vi "gyro -- async pll monitor V1.vi"(8 "pll engine pair IN":T6, 11 "pll monitor event pair IN":T6) -> ()   [LabVIEW 2020]
uses:
  lorentzian.ctl
  circle corners.ctl
  show-win- control.ctl
  server talk-to-back pair.ctl
  server talkback message type.ctl
  server talkto message type.ctl
  pll internal user event action.ctl
  launch items list.ctl
  que event bag action.ctl
  agregator -- action.ctl
  publisher action.ctl
  cursor action.ctl
  four-corner circle transformation.ctl
  draw a circle.vi
  draw a complex arrow.vi
  Q -- check range -- i -- real.vi
  generate linear region.vi
  draw a complex line.vi
  Q - not nan -- real.vi
panel:
  out "slow G (Hz)":dbl=24.16832544290019 format="%#.4f"
  out "slow f (Hz)":dbl=46363.51241324636 format="%#.11f"
  in  "all 3":T1(tab)
  in  "Reset lore :q":bool
  in  "Tab Control":enum32{"PID", "hist", "params"}(tab)
  out "Plot: complex plane":cluster{dbl[], dbl[]}[](graph)
  out "Plot: complex- hist":cluster{dbl[], dbl[]}[](graph)=[{[-9.526305317469014e-05, -9.526305317469014e-05, -9.526305317469014e-05, -9.526305317469014e-05, -9.526305317469014e-05, -9.526305317469014e-05, -9.526305317469014e-05, -9.526305317469014e-05, -9.526305317469014e-05, -9.526305317469014e-05, -9.526305317469014e-05, -9.526305317469014e-05, -9.496573362823372e-05, -9.462272279446522e-05, -9.456910422622903e-05, -9.455599564968666e-05, -9.455599564968666e-05, -9.455599564968666e-05, -9.455599564968666e-05, -9.455599564968666e-05, -9.455599564968666e-05, -9.530610879315279e-05, -9.530610879315279e-05, -9.634850628222362e-05, -9.634850628222362e-05, -9.634850628222362e-05, -9.634850628222362e-05, -9.634850628222362e-05, -9.634850628222362e-05, -9.634850628222362e-05, -0.00010067313796781224, -0.00010168181201432396, -0.00010343088718200523, -0.00010398871218266516, -0.00010398871218266516, -0.00010398871218266516, -0.00010398871218266516, -0.00010398871218266516, -0.00010398871218266516, -0.00010398871218266516, -0.00010398871218266516, -0.00010398871218266516, -0.00011483545491618031, -0.00011483545491618031, -0.00011483545491618031, -0.00011483545491618031, -0.00011483545491618031, -0.00011483545491618031, -0.00011483545491618031, -0.00011483545491618031], [7.970920146417072e-05, 7.970920146417072e-05, 7.970920146417072e-05, 7.970920146417072e-05, 7.970920146417072e-05, 7.970920146417072e-05, 7.970920146417072e-05, 7.970920146417072e-05, 7.970920146417072e-05, 7.970920146417072e-05, 7.970920146417072e-05, 7.970920146417072e-05, 7.992857617299889e-05, 8.004706678063113e-05, 8.0440222108718e-05, 8.032807976592085e-05, 8.032807976592085e-05, 8.032807976592085e-05, 8.032807976592085e-05, 8.032807976592085e-05, 8.032807976592085e-05, 8.12855651877623e-05, 8.12855651877623e-05, 8.097547218826884e-05, 8.097547218826884e-05, 8.097547218826884e-05, 8.097547218826884e-05, 8.097547218826884e-05, 8.097547218826884e-05, 8.097547218826884e-05, 8.470777605978184e-05, 8.527717057334149e-05, 8.650804581518505e-05, 8.815252786351578e-05, 8.815252786351578e-05, 8.815252786351578e-05, 8.815252786351578e-05, 8.815252786351578e-05, 8.815252786351578e-05, 8.815252786351578e-05, 8.815252786351578e-05, 8.815252786351578e-05, 9.872168338494033e-05, 9.872168338494033e-05, 9.872168338494033e-05, 9.872168338494033e-05, 9.872168338494033e-05, 9.872168338494033e-05, 9.872168338494033e-05, 9.872168338494033e-05]}, {[3.818876044553316e-06, 3.7612071619776832e-06, 3.588301685066841e-06, 3.300462948780953e-06, 2.8981959200717497e-06, 2.3822063119988216e-06, 1.7533993456691853e-06, 1.0128781621718285e-06, 1.6194188729338013e-07, -7.979166475899173e-07, -1.8650135244457675e-06, -3.037476692750206e-06, -4.313249253700366e-06, -5.690093068713917e-06, -7.1655926858846405e-06, -8.737159577505894e-06, -1.0402036681227744e-05, -1.2157303236881222e-05, -1.3999879910484142e-05, -1.592653419643923e-05, -1.79338860884474e-05, -2.001841400918731e-05, -2.2176460988358644e-05, -2.440424107825063e-05, -2.6697845995580853e-05, -2.9053251977952116e-05, -3.146632684289902e-05, -3.3932837237140076e-05, -3.6448456063317944e-05, -3.900877007119849e-05, -4.1609287600011325e-05, -4.4245446458349125e-05, -4.691262192780158e-05, -4.9606134876282945e-05, -5.232125996681972e-05, -5.505323394739742e-05, -5.779726400732312e-05, -6.054853618544401e-05, -6.330222381547109e-05, -6.605349599359198e-05, -6.879752605351768e-05, -7.152950003409537e-05, -7.424462512463216e-05, -7.693813807311352e-05, -7.960531354256597e-05, -8.224147240090377e-05, -8.484198992971662e-05, -8.740230393759715e-05, -8.991792276377502e-05, -9.238443315801609e-05, -9.479750802296298e-05, -9.715291400533426e-05, -9.944651892266448e-05, -0.00010167429901255647, -0.00010383234599172779, -0.00010591687391246771, -0.00010792422580447587, -0.00010985088009043097, -0.00011169345676403388, -0.00011344872331968736, -0.00011511360042340923, -0.00011668516731503045, -0.00011816066693220119, -0.00011953751074721475, -0.0001208132833081649, -0.00012198574647646935, -0.0001230528433533252, -0.0001240127018882085, -0.00012486363816308695, -0.0001256041593465843, -0.00012623296631291396, -0.00012674895592098688, -0.00012715122294969607, -0.00012743906168598198, -0.00012761196716289282, -0.00012766963604546842, -0.00012761196716289282, -0.00012743906168598198, -0.00012715122294969607, -0.00012674895592098688, -0.00012623296631291396, -0.00012560415934658432, -0.00012486363816308695, -0.00012401270188820853, -0.00012305284335332523, -0.00012198574647646936, -0.00012081328330816493, -0.00011953751074721476, -0.00011816066693220122, -0.00011668516731503051, -0.00011511360042340925, -0.00011344872331968739, -0.0001116934567640339, -0.000109850880090431, -0.00010792422580447591, -0.00010591687391246773, -0.00010383234599172784, -0.0001016742990125565, -9.944651892266452e-05, -9.715291400533429e-05, -9.479750802296303e-05, -9.238443315801612e-05, -8.991792276377506e-05, -8.740230393759719e-05, -8.484198992971665e-05, -8.22414724009038e-05, -7.9605313542566e-05, -7.69381380731136e-05, -7.424462512463222e-05, -7.152950003409544e-05, -6.879752605351773e-05, -6.605349599359204e-05, -6.330222381547115e-05, -6.054853618544405e-05, -5.779726400732316e-05, -5.505323394739747e-05, -5.232125996681976e-05, -4.960613487628297e-05, -4.691262192780161e-05, -4.424544645834915e-05, -4.160928760001134e-05, -3.900877007119856e-05, -3.644845606331801e-05, -3.393283723714014e-05, -3.146632684289907e-05, -2.905325197795217e-05, -2.66978459955809e-05, -2.4404241078250677e-05, -2.2176460988358678e-05, -2.0018414009187342e-05, -1.7933886088447427e-05, -1.5926534196439257e-05, -1.3999879910484162e-05, -1.2157303236881242e-05, -1.0402036681227757e-05, -8.7371595775059e-06, -7.165592685884681e-06, -5.690093068713951e-06, -4.3132492537004e-06, -3.037476692750233e-06, -1.8650135244457946e-06, -7.979166475899309e-07, 1.6194188729336657e-07, 1.012878162171815e-06, 1.7533993456691853e-06, 2.3822063119988216e-06, 2.8981959200717497e-06, 3.300462948780953e-06, 3.588301685066841e-06, 3.7612071619776832e-06], [0.00013328633245229232, 0.00013603941615311703, 0.0001387876700096264, 0.0001415262726506931, 0.00014425041963670132, 0.00014695533188816622, 0.0001496362640698634, 0.00015228851291575925, 0.00015490742548013788, 0.00015748840730044888, 0.00016002693045755594, 0.0001625185415192455, 0.0001649588693530602, 0.00016734363279475065, 0.00016966864815889197, 0.00017192983657849, 0.00017412323116069973, 0.00017624498394610346, 0.00017829137265933922, 0.00018025880723923637, 0.00018214383613700304, 0.00018394315237141542, 0.0001856535993303866, 0.00018727217630873675, 0.00018879604377244967, 0.0001902225283401804, 0.0001915491274732744, 0.0001927735138660708, 0.00019389353952878736, 0.00019490723955582442, 0.00019581283557287696, 0.00019660873885680747, 0.00019729355312280615, 0.00019786607697394902, 0.00019832530600885628, 0.0001986704345837536, 0.00019890085722584514, 0.00019901616969551854, 0.00019901616969551854, 0.00019890085722584514, 0.0001986704345837536, 0.00019832530600885628, 0.00019786607697394902, 0.00019729355312280615, 0.00019660873885680747, 0.00019581283557287696, 0.00019490723955582442, 0.0001938935395287874, 0.00019277351386607082, 0.0001915491274732744, 0.0001902225283401804, 0.00018879604377244967, 0.00018727217630873675, 0.00018565359933038662, 0.00018394315237141545, 0.00018214383613700307, 0.00018025880723923637, 0.00017829137265933922, 0.00017624498394610348, 0.00017412323116069973, 0.00017192983657849, 0.000169668648158892, 0.00016734363279475065, 0.00016495886935306023, 0.00016251854151924552, 0.00016002693045755596, 0.0001574884073004489, 0.00015490742548013788, 0.00015228851291575928, 0.00014963626406986344, 0.00014695533188816625, 0.00014425041963670135, 0.00014152627265069312, 0.0001387876700096264, 0.00013603941615311706, 0.00013328633245229235, 0.00013053324875146764, 0.0001277849948949583, 0.00012504639225389158, 0.00012232224526788335, 0.00011961733301641843, 0.00011693640083472126, 0.00011428415198882542, 0.0001116652394244468, 0.00010908425760413579, 0.00010654573444702874, 0.00010405412338533918, 0.00010161379555152444, 9.922903210983402e-05, 9.69040167456927e-05, 9.464282832609468e-05, 9.244943374388495e-05, 9.032768095848119e-05, 8.828129224524545e-05, 8.631385766534829e-05, 8.44288287675816e-05, 8.262951253316924e-05, 8.091906557419806e-05, 7.930048859584792e-05, 7.777662113213499e-05, 7.635013656440427e-05, 7.502353743131027e-05, 7.379915103851385e-05, 7.267912537579728e-05, 7.166542534876021e-05, 7.07598293317077e-05, 6.996392604777719e-05, 6.927911178177851e-05, 6.870658793063563e-05, 6.824735889572837e-05, 6.790223032083105e-05, 6.76718076787395e-05, 6.755649520906611e-05, 6.755649520906611e-05, 6.76718076787395e-05, 6.790223032083104e-05, 6.824735889572836e-05, 6.870658793063562e-05, 6.92791117817785e-05, 6.996392604777719e-05, 7.075982933170768e-05, 7.166542534876019e-05, 7.267912537579724e-05, 7.379915103851382e-05, 7.502353743131023e-05, 7.635013656440423e-05, 7.777662113213495e-05, 7.930048859584787e-05, 8.091906557419801e-05, 8.262951253316918e-05, 8.442882876758158e-05, 8.631385766534825e-05, 8.828129224524542e-05, 9.032768095848116e-05, 9.244943374388492e-05, 9.464282832609465e-05, 9.690401674569261e-05, 9.922903210983394e-05, 0.00010161379555152437, 0.00010405412338533911, 0.00010654573444702866, 0.00010908425760413571, 0.00011166523942444672, 0.00011428415198882535, 0.0001169364008347212, 0.00011961733301641839, 0.0001223222452678833, 0.00012504639225389153, 0.00012778499489495826, 0.0001305332487514676]}, {[3.628480178228017e-06, -3.271926156370463e-06, -1.0172332490968943e-05, -1.7072738825567422e-05, -2.3973145160165903e-05, -3.087355149476438e-05, -3.777395782936286e-05, -4.467436416396134e-05, -5.157477049855982e-05, -5.8475176833158303e-05, -6.537558316775678e-05, -7.227598950235527e-05, -7.917639583695374e-05, -8.607680217155223e-05, -9.29772085061507e-05, -9.987761484074919e-05, -0.00010677802117534766, -0.00011367842750994615, -0.00012057883384454462, -0.00012747924017914312], [0.00013828619430891303, 0.0001377598930608477, 0.00013723359181278235, 0.00013670729056471703, 0.00013618098931665167, 0.00013565468806858635, 0.000135128386820521, 0.00013460208557245567, 0.00013407578432439034, 0.00013354948307632499, 0.00013302318182825966, 0.0001324968805801943, 0.00013197057933212898, 0.00013144427808406365, 0.0001309179768359983, 0.00013039167558793297, 0.00012986537433986762, 0.0001293390730918023, 0.00012881277184373694, 0.00012828647059567161]}, {[-0.00012747924017914312, -0.0001271379440244435, -0.00012679664786974387, -0.00012645535171504425, -0.00012611405556034463, -0.00012577275940564502, -0.00012543146325094537, -0.00012509016709624576, -0.00012474887094154614, -0.00012440757478684653, -0.00012406627863214688, -0.00012372498247744727, -0.00012338368632274765, -0.00012304239016804804, -0.0001227010940133484, -0.00012235979785864878, -0.00012201850170394916, -0.00012167720554924953, -0.00012133590939454991, -0.00012099461323985029], [0.00012828647059567161, 0.00012822947554103566, 0.0001281724804863997, 0.00012811548543176373, 0.00012805849037712778, 0.00012800149532249183, 0.00012794450026785587, 0.00012788750521321992, 0.00012783051015858394, 0.000127773515103948, 0.00012771652004931204, 0.0001276595249946761, 0.0001276025299400401, 0.00012754553488540416, 0.0001274885398307682, 0.00012743154477613225, 0.0001273745497214963, 0.00012731755466686032, 0.00012726055961222437, 0.00012720356455758842]}, {[-0.00012747924017914312, -0.00012715053574649993, -0.0001268218313138567, -0.0001264931268812135, -0.00012616442244857027, -0.00012583571801592707, -0.00012550701358328385, -0.00012517830915064065, -0.00012484960471799742, -0.00012452090028535422, -0.00012419219585271102, -0.0001238634914200678, -0.0001235347869874246, -0.00012320608255478137, -0.00012287737812213817, -0.00012254867368949494, -0.00012221996925685174, -0.00012189126482420853, -0.00012156256039156532, -0.0001212338559589221], [0.00012828647059567161, 0.00012839456729972132, 0.00012850266400377103, 0.0001286107607078207, 0.00012871885741187042, 0.00012882695411592013, 0.00012893505081996984, 0.00012904314752401955, 0.00012915124422806923, 0.00012925934093211894, 0.00012936743763616865, 0.00012947553434021836, 0.00012958363104426804, 0.00012969172774831775, 0.00012979982445236746, 0.00012990792115641716, 0.00013001601786046687, 0.00013012411456451655, 0.00013023221126856626, 0.00013034030797261597]}, {[-6.692524185707827e-05, -6.639894060901293e-05, -6.587263936094759e-05, -6.534633811288225e-05, -6.482003686481692e-05, -6.429373561675158e-05, -6.376743436868624e-05, -6.32411331206209e-05, -6.271483187255556e-05, -6.218853062449022e-05, -6.16622293764249e-05, -6.113592812835956e-05, -6.060962688029422e-05, -6.008332563222888e-05, -5.955702438416354e-05, -5.9030723136098205e-05, -5.8504421888032865e-05, -5.7978120639967525e-05, -5.745181939190219e-05, -5.692551814383685e-05], [0.0001988401926309779, 0.0001919397862963794, 0.00018503937996178094, 0.00017813897362718245, 0.00017123856729258396, 0.00016433816095798548, 0.00015743775462338702, 0.00015053734828878853, 0.00014363694195419004, 0.00013673653561959158, 0.0001298361292849931, 0.0001229357229503946, 0.00011603531661579613, 0.00010913491028119764, 0.00010223450394659917, 9.533409761200068e-05, 8.843369127740221e-05, 8.153328494280372e-05, 7.463287860820525e-05, 6.773247227360676e-05]}, {[-5.692551814383685e-05, -5.686852308920089e-05, -5.681152803456494e-05, -5.675453297992898e-05, -5.669753792529302e-05, -5.6640542870657065e-05, -5.658354781602111e-05, -5.6526552761385154e-05, -5.6469557706749195e-05, -5.6412562652113236e-05, -5.6355567597477284e-05, -5.6298572542841325e-05, -5.6241577488205367e-05, -5.618458243356941e-05, -5.6127587378933456e-05, -5.60705923242975e-05, -5.601359726966154e-05, -5.595660221502558e-05, -5.589960716038963e-05, -5.584261210575367e-05], [6.773247227360675e-05, 6.807376842830637e-05, 6.841506458300599e-05, 6.875636073770562e-05, 6.909765689240524e-05, 6.943895304710487e-05, 6.978024920180448e-05, 7.012154535650411e-05, 7.046284151120373e-05, 7.080413766590336e-05, 7.114543382060297e-05, 7.14867299753026e-05, 7.182802613000222e-05, 7.216932228470185e-05, 7.251061843940146e-05, 7.28519145941011e-05, 7.319321074880071e-05, 7.353450690350034e-05, 7.387580305819996e-05, 7.421709921289959e-05]}, {[-5.692551814383685e-05, -5.7033614847886554e-05, -5.7141711551936256e-05, -5.724980825598596e-05, -5.7357904960035666e-05, -5.746600166408537e-05, -5.757409836813507e-05, -5.768219507218477e-05, -5.7790291776234474e-05, -5.7898388480284176e-05, -5.8006485184333885e-05, -5.811458188838359e-05, -5.822267859243329e-05, -5.833077529648299e-05, -5.843887200053269e-05, -5.8546968704582395e-05, -5.86550654086321e-05, -5.8763162112681805e-05, -5.887125881673151e-05, -5.897935552078121e-05], [6.773247227360675e-05, 6.806117670624996e-05, 6.838988113889317e-05, 6.871858557153638e-05, 6.90472900041796e-05, 6.93759944368228e-05, 6.970469886946601e-05, 7.003340330210922e-05, 7.036210773475244e-05, 7.069081216739565e-05, 7.101951660003886e-05, 7.134822103268207e-05, 7.167692546532529e-05, 7.20056298979685e-05, 7.233433433061171e-05, 7.266303876325491e-05, 7.299174319589813e-05, 7.332044762854134e-05, 7.364915206118455e-05, 7.397785649382777e-05]}, {[-6.3712435350134095e-06, -5.318641038882734e-06, -4.266038542752058e-06, -3.213436046621383e-06, -2.160833550490707e-06, -1.1082310543600322e-06, -5.56285582293566e-08, 9.96973937901319e-07, 2.0495764340319955e-06, 3.1021789301626703e-06, 4.154781426293345e-06, 5.2073839224240215e-06, 6.259986418554696e-06, 7.312588914685373e-06, 8.365191410816048e-06, 9.417793906946724e-06, 1.04703964030774e-05, 1.1522998899208077e-05, 1.257560139533875e-05, 1.3628203891469427e-05], [0.00026939391466628416, 0.0002555931019970872, 0.00024179228932789024, 0.0002279914766586933, 0.00021419066398949631, 0.00020038985132029937, 0.00018658903865110242, 0.00017278822598190544, 0.00015898741331270847, 0.00014518660064351152, 0.00013138578797431457, 0.0001175849753051176, 0.00010378416263592065, 8.998334996672367e-05, 7.618253729752673e-05, 6.238172462832975e-05, 4.85809119591328e-05, 3.478009928993583e-05, 2.097928662073888e-05, 7.178473951541904e-06]}, {[1.3628203891469427e-05, 1.374219400074134e-05, 1.3856184110013255e-05, 1.397017421928517e-05, 1.4084164328557083e-05, 1.4198154437828998e-05, 1.4312144547100912e-05, 1.4426134656372826e-05, 1.454012476564474e-05, 1.4654114874916653e-05, 1.4768104984188567e-05, 1.4882095093460481e-05, 1.4996085202732395e-05, 1.511007531200431e-05, 1.5224065421276224e-05, 1.5338055530548138e-05, 1.5452045639820052e-05, 1.5566035749091966e-05, 1.568002585836388e-05, 1.5794015967635795e-05], [7.178473951541904e-06, 7.861066260941151e-06, 8.543658570340397e-06, 9.226250879739644e-06, 9.90884318913889e-06, 1.0591435498538137e-05, 1.1274027807937384e-05, 1.195662011733663e-05, 1.2639212426735877e-05, 1.3321804736135124e-05, 1.400439704553437e-05, 1.4686989354933617e-05, 1.5369581664332864e-05, 1.605217397373211e-05, 1.6734766283131355e-05, 1.7417358592530604e-05, 1.809995090192985e-05, 1.87825432113291e-05, 1.9465135520728344e-05, 2.014772783012759e-05]}, {[1.3628203891469427e-05, 1.3412010483370021e-05, 1.3195817075270614e-05, 1.2979623667171208e-05, 1.2763430259071802e-05, 1.2547236850972395e-05, 1.233104344287299e-05, 1.2114850034773584e-05, 1.1898656626674176e-05, 1.1682463218574771e-05, 1.1466269810475365e-05, 1.1250076402375958e-05, 1.1033882994276552e-05, 1.0817689586177147e-05, 1.0601496178077741e-05, 1.0385302769978334e-05, 1.0169109361878928e-05, 9.95291595377952e-06, 9.736722545680117e-06, 9.52052913758071e-06], [7.178473951541904e-06, 7.835882816828328e-06, 8.49329168211475e-06, 9.150700547401175e-06, 9.8081094126876e-06, 1.0465518277974024e-05, 1.1122927143260446e-05, 1.178033600854687e-05, 1.2437744873833295e-05, 1.3095153739119718e-05, 1.3752562604406142e-05, 1.4409971469692566e-05, 1.506738033497899e-05, 1.5724789200265415e-05, 1.6382198065551837e-05, 1.703960693083826e-05, 1.7697015796124686e-05, 1.8354424661411112e-05, 1.901183352669753e-05, 1.9669242391983957e-05]}]
  out "fast G (Hz)":dbl=23.890697353762498 format="%#.4f"
  in  "Reset freq :r":bool
  in  "lorentzian":T2={"A (VHz)"=0.0013732658487984977, "f (Hz)"=46364.101188801076, "G (Hz)"=24.052820242417244, "phi(rad)"=4.682548985119491, "Q"=1927.5952142625588, "Norm  Ampl"=nan, "bg (V)"=9.232975216617241e-07+0.00011328685513440606i, "4corners"={"z (-pi/2)"=-5.784846603575453e-05+5.7921940748033466e-05i, "z(inf)"=9.232975216617241e-07+0.00011328685513440606i, "z (pi/2)"=-5.444161686471088e-05+0.00017205861869182233i, "z center"=-5.61450414502327e-05+0.00011499027971992789i, "z(0)"=-0.00011321338042212712+0.00011669370430544972i, "radius"=5.709375594869902e-05}} {"bg (V)" format="%#9_9f"; "Q" format="%#9_9f"; "phi(rad)" format="%#9_9f"; "G (Hz)" format="%#9_9f"; "f (Hz)" format="%#9_9f"}
  in  "Toggle PLL :@":bool
  out "fast f (Hz)":dbl=46363.6845772732 format="%#.11f"
  in  "PLL is ON":bool
  in  "publish dt (sec)":dbl=0.01 format="%#_10f"
  in  "average time (sec)":dbl=2.0 format="%#_10f"
  in  "lorentzian -- basic":T2={"A (VHz)"=1.0, "f (Hz)"=1000.0, "G (Hz)"=3.0, "phi(rad)"=0.0, "Q"=300.0, "Norm  Ampl"=nan, "bg (V)"=0.0+0.0i, "4corners"={"z (-pi/2)"=9.277908004825974e-07+0.0007240755403629966i, "z(inf)"=2.6527949823343002e-05+0.0007477540585896028i, "z (pi/2)"=2.8494315967368497e-06+0.0007733542176124632i, "z center"=1.8886111986097237e-06+0.0007487148789877299i, "z(0)"=-2.2750727426123552e-05+0.000749675699385857i, "radius"=2.4658065287076567e-05}} {"bg (V)" format="%#9_9f"; "Q" format="%#9_9f"; "phi(rad)" format="%#9_9f"; "G (Hz)" format="%#9_9f"; "f (Hz)" format="%#9_9f"}
  in  "save lor for later":bool
  in  "reset from basic":bool
  out "zi out Im (V)":dbl=0.00011062417845810371 format="%#.8f"
  out "zi out Re (V)":dbl=-0.00011339640178767734 format="%#.8f"
  out "publish message":T4={"freq (Hz)"=46363.51241324636, "gamma (Hz)"=24.16832544290019, "Voltage (V)"=-0.00011339640178767734+0.00011062417845810371i}
  out "zi out (V)":cdb=-0.00011339640178767734+0.00011062417845810371i
  out "is publish loop stoped?":bool=TRUE
  out "window":T5={"cen (Hz)"=45496.74569300777, "win (Hz)"=29.962105514646385, "left (Hz)"=45481.76464025045, "right (Hz)"=45511.72674576509}
  out "running lorentzian out":T2={"A (VHz)"=0.0013788688861127354, "f (Hz)"=46363.6845772732, "G (Hz)"=23.890697353762498, "phi(rad)"=4.689952869394783, "Q"=1921.793640717071, "Norm  Ampl"=nan, "bg (V)"=1.441663885059972e-06+0.00010805339490546445i, "4corners"={"z (-pi/2)"=-4.886429450544085e-05+0.00017233029636879173i, "z(inf)"=1.441663885059972e-06+0.00010805339490546445i, "z (pi/2)"=-6.283523757826731e-05+5.7747436514963635e-05i, "z center"=-5.584976604185408e-05+0.00011503886644187768i, "z(0)"=-0.00011314119596876813+0.00012202433797829091i, "radius"=5.771572364318533e-05}} {"bg (V)" format="%#9_9f"; "Q" format="%#9_9f"; "phi(rad)" format="%#9_9f"; "G (Hz)" format="%#9_9f"; "f (Hz)" format="%#9_9f"}
  in  "lorentzian -- hist":T2={"A (VHz)"=0.00200421395131866, "f (Hz)"=46345.85168996005, "G (Hz)"=30.48500465115163, "phi(rad)"=-1.4946726575691582, "Q"=1520.2835695880153, "Norm  Ampl"=nan, "bg (V)"=3.628480178228017e-06+0.00013828619430891303i, "4corners"={"z (-pi/2)"=-6.692524185707827e-05+0.0001988401926309779i, "z(inf)"=3.628480178228017e-06+0.00013828619430891303i, "z (pi/2)"=-5.692551814383685e-05+6.773247227360675e-05i, "z center"=-6.192538000045756e-05+0.00013328633245229232i, "z(0)"=-0.00012747924017914312+0.00012828647059567161i, "radius"=6.574425604501088e-05}} {"bg (V)" format="%#9_9f"; "Q" format="%#9_9f"; "phi(rad)" format="%#9_9f"; "G (Hz)" format="%#9_9f"; "f (Hz)" format="%#9_9f"}
  out "static lorentzian out":T2={"A (VHz)"=0.0013732658487984977, "f (Hz)"=46364.101188801076, "G (Hz)"=24.052820242417244, "phi(rad)"=4.682548985119491, "Q"=1927.5952142625588, "Norm  Ampl"=nan, "bg (V)"=9.232975216617241e-07+0.00011328685513440606i, "4corners"={"z (-pi/2)"=-5.784846603575453e-05+5.7921940748033466e-05i, "z(inf)"=9.232975216617241e-07+0.00011328685513440606i, "z (pi/2)"=-5.444161686471088e-05+0.00017205861869182233i, "z center"=-5.61450414502327e-05+0.00011499027971992789i, "z(0)"=-0.00011321338042212712+0.00011669370430544972i, "radius"=5.709375594869902e-05}} {"bg (V)" format="%#9_9f"; "Q" format="%#9_9f"; "phi(rad)" format="%#9_9f"; "G (Hz)" format="%#9_9f"; "f (Hz)" format="%#9_9f"}
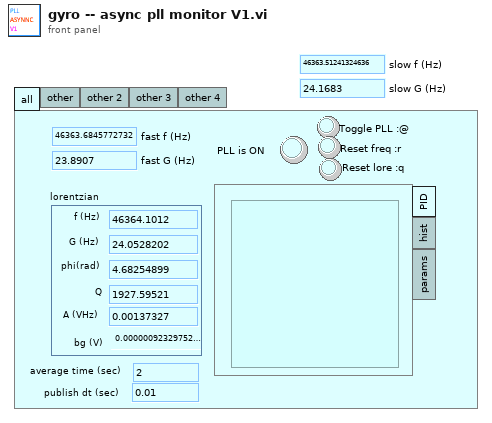
[diagram p1: front panel]
types:
  T1 = enum32{"all", "other", "other 2", "other 3", "other 4"}
  T2 = typedef "lorentzian.ctl" = cluster{"A (VHz)":dbl, "f (Hz)":dbl, "G (Hz)":dbl, "phi(rad)":dbl, "Q":dbl, "Norm  Ampl":dbl, "bg (V)":cdb, "4corners":T3}
  T3 = typedef "circle corners.ctl" = cluster{"z (-pi/2)":cdb, "z(inf)":cdb, "z (pi/2)":cdb, "z center":cdb, "z(0)":cdb, "radius":dbl}
  T4 = cluster{"freq (Hz)":dbl, "gamma (Hz)":dbl, "Voltage (V)":cdb}
  T5 = typedef "show-win- control.ctl" = cluster{"cen (Hz)":dbl, "win (Hz)":dbl, "left (Hz)":dbl, "right (Hz)":dbl}
  T6 = typedef "server talk-to-back pair.ctl" = cluster{"talkback event":refnum<user-event>, "talkto event":refnum<user-event>}
  T7 = typedef "agregator -- action.ctl" = enum16{"append", "interpolate", "empty!", "force", "init", "scale", "read last"}
  T8 = typedef "launch items list.ctl" = enum16{"void", "source", "pll engine", "pll monitor", "sweeper engine", "sweeper monitor", "fitter", "--Keys"}
  T9 = typedef "que event bag action.ctl" = enum16{"check", "add", "init"}
  T10 = typedef "pll internal user event action.ctl" = enum16{"gear pll engine", "start pll async", "stop pll async", "toggle pll async", "gear sweeper", "start sweeper", "stop sweeper", "toggle sweeper", "accept frequency", "reset lorentzian", "accept lorentzian", "update cursors", "pause pll", "unpause pll", "void", "exit", "gear sweeper monitor", "gear sweeper engine", "gear fitter", "gear sourcer", "gear pll monitor"}
  T11 = enum16{"stop", "start", "update pars", "update request", "new", "launch", "exit", "get", "reset", "pause", "unpause"}
  T12 = typedef "cursor action.ctl" = enum16{"range", "read", "write", "check", "zoom out", "smart zoom out", "zoom to aspect ratio 1", "zoom to win", "zoom out 20%", "zoom in 20%", "-empty", "smart zoom out&aspect", "move range left 20%", "move range right 20%", "move range up 20%", "move range down 20%", "zoom to X win", "zoom to Y win", "zoom out X", "zoom out Y", "zoom in X", "zoom in Y", "check plot scale"}
  T13 = typedef "four-corner circle transformation.ctl" = enum16{"z(c) z(inf)", "z(c) z(zero)", "fix phase", "calculate lorentzian", "z(0) z(+-pi/2)", "shift to zcenter", "to  canonical", "get canonical phase", "get4corners", "update lorentzian -- from z0", "fake gamma normal", "fake gamma heat", "calculate complex slope", "get f0 given f and phi"}
  T14 = typedef "eventvkey.ctl" = enum16{"ASCII", "Enter", "Return", "Shift", "Ctrl", "Alt", "Cmd", "Opt", "Caps", "NumLock", "Clear", "Break", "Up", "Down", "Left", "Right", "Insert", "Delete", "Home", "End", "PageUp", "PageDown", "Escape", "Help", "Pause", "ScrollLock", "F1", "F2", "F3", "F4", "F5", "F6", "F7", "F8", "F9", "F10", "F11", "F12", "F13", "F14", "F15", "F16", "F17", "F18", "F19", "F20", "F21", "F22", "F23", "F24", "Play", "VolumeUp", "VolumeDown", "Mute", "Two Byte Char"}
  T15 = typedef "publisher action.ctl" = enum16{"set", "get", "init", "check"}
  T16 = typedef "server talkto message type.ctl" = cluster{"message":enum16{"stop", "start", "update pars", "update request", "new", "launch", "exit", "get", "reset", "pause", "unpause"}}
  T17 = typedef "pll talkback data type.ctl" = cluster{"freq (Hz)":dbl, "gamma (Hz)":dbl, "Voltage (V)":cdb, "overlimit ?":bool, "running lorentzian out":T2, "static lorentzian out":T2}
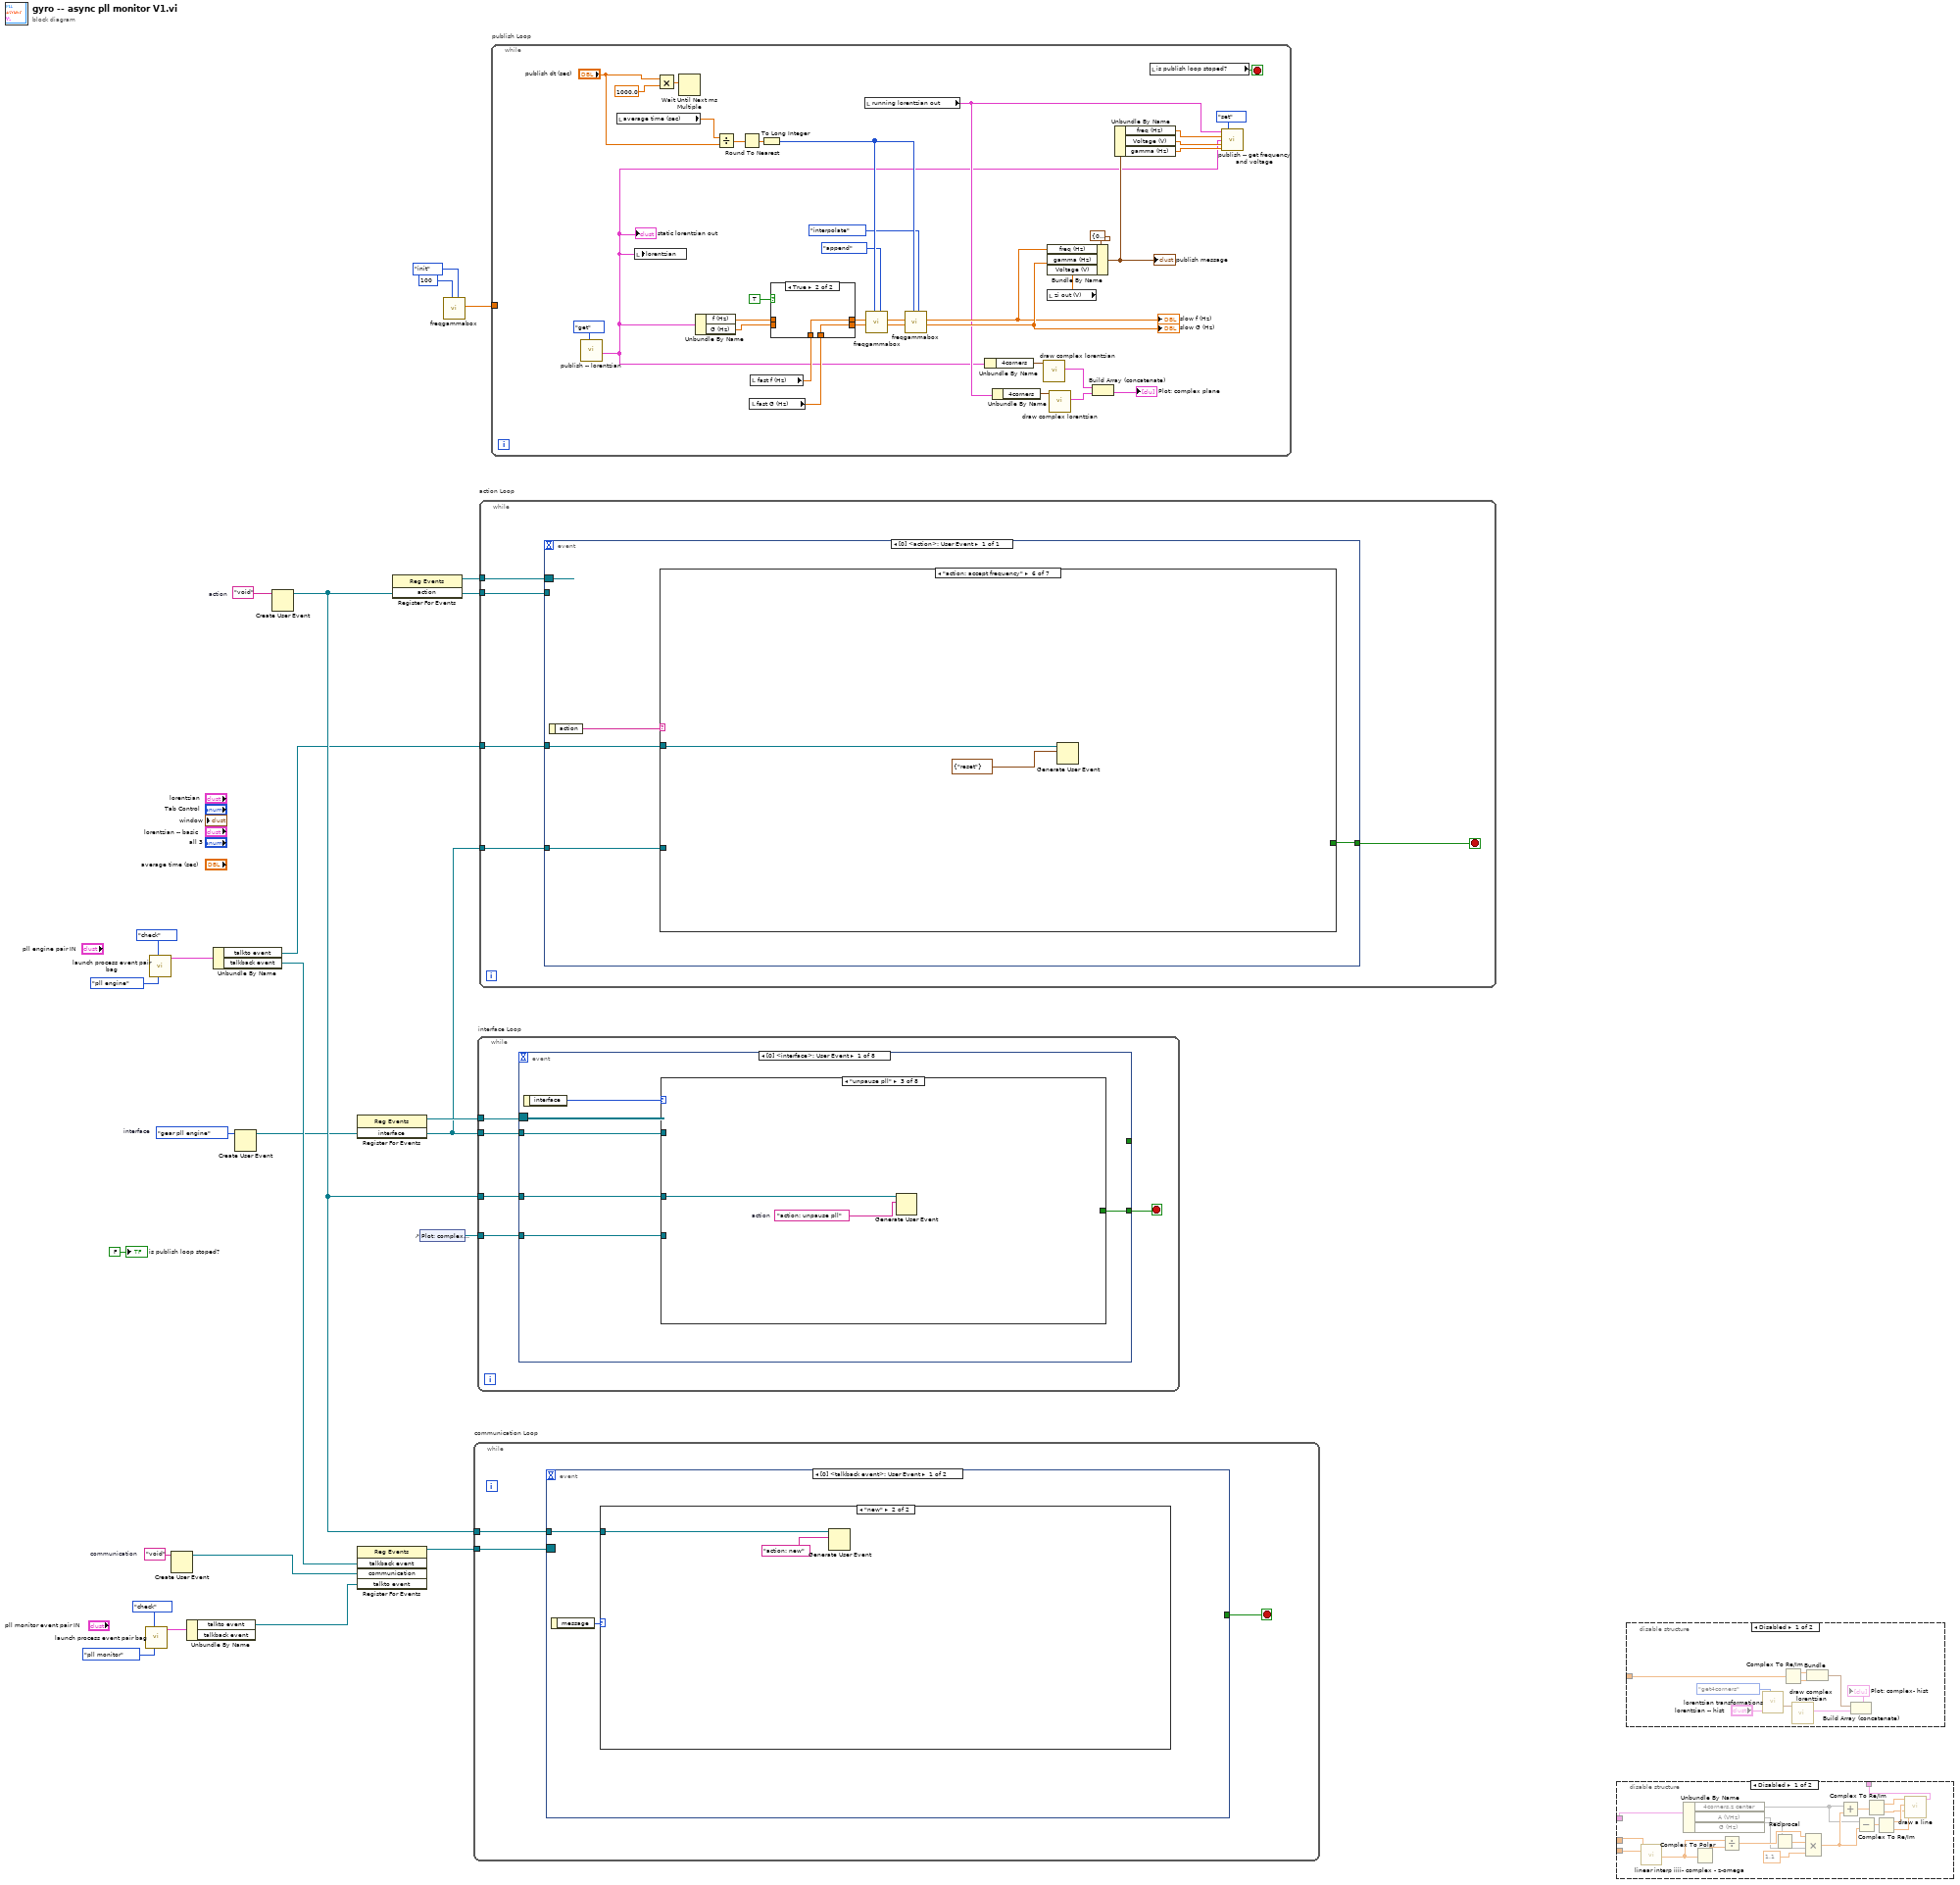
[diagram p0: block diagram]
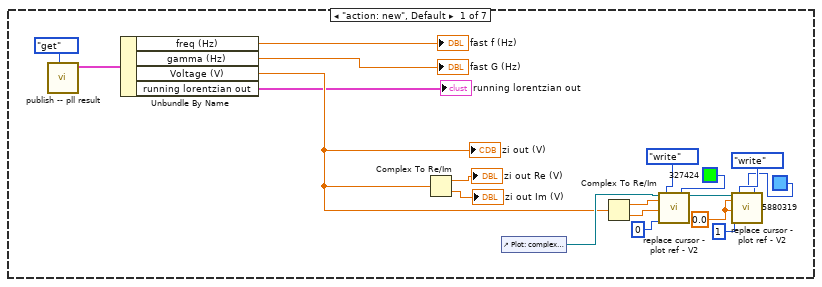
[diagram p4: hidden frame]
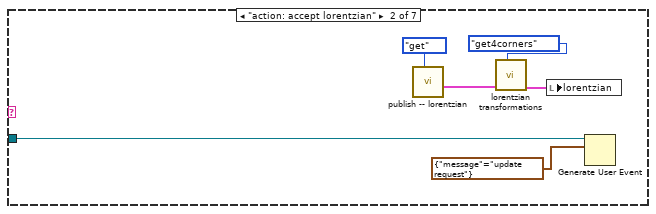
[diagram p5: hidden frame]
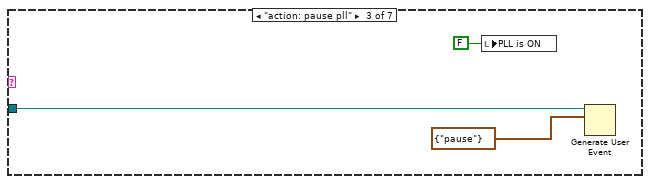
[diagram p6: hidden frame]
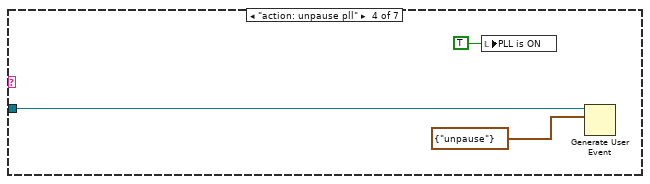
[diagram p7: hidden frame]
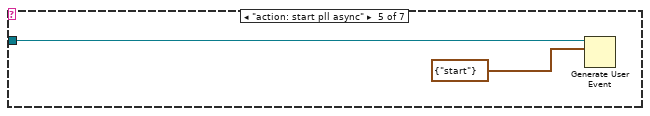
[diagram p8: hidden frame]
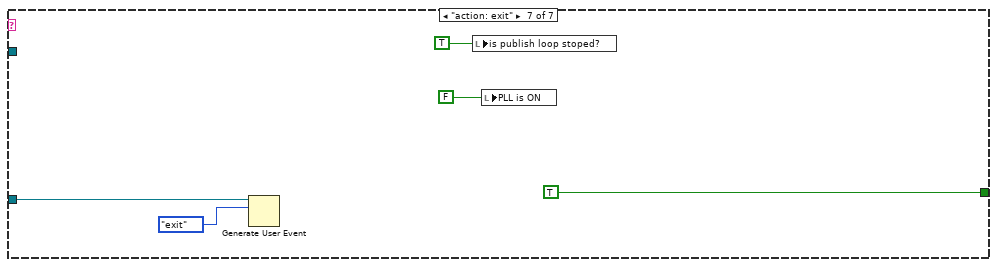
[diagram p9: hidden frame]
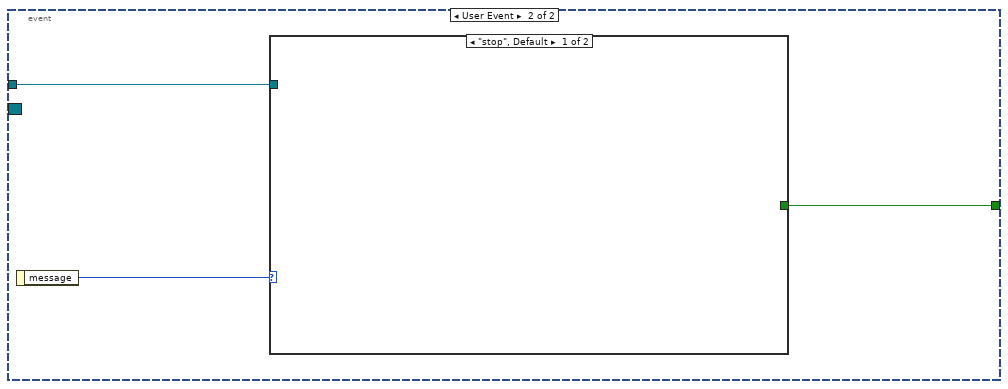
[diagram p12: hidden frame]
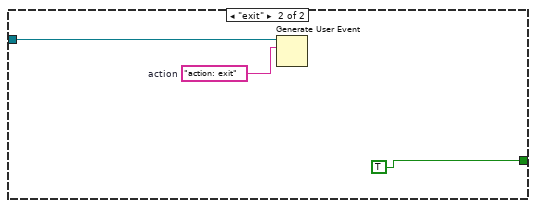
[diagram p13: hidden frame]
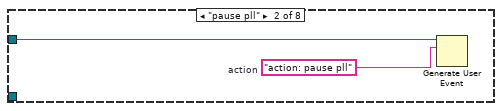
[diagram p15: hidden frame]
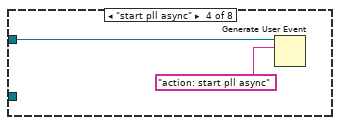
[diagram p16: hidden frame]
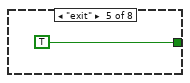
[diagram p17: hidden frame]
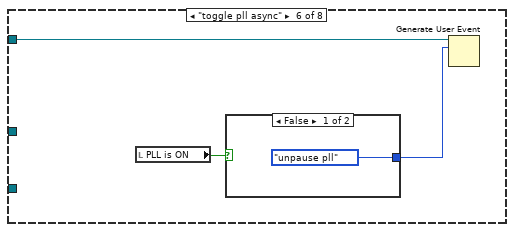
[diagram p18: hidden frame]
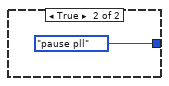
[diagram p19: hidden frame]
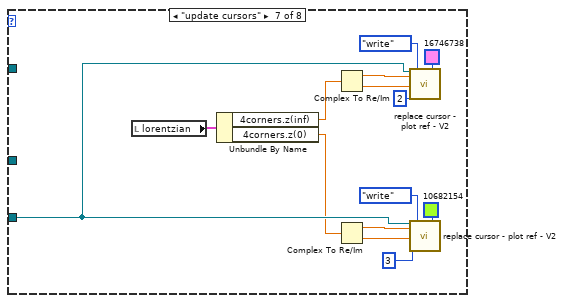
[diagram p20: hidden frame]
diagram:
  w16 = "void"  # communication
  w18 = "void"  # action
  w20 = pll_internal_user_event_action."gear pll engine"  # interface
  n1 = call "launch process event pair bag.vi"("launch items"=launch_items_list."pll monitor", "bag action"=que_event_bag_action."check") -> ("even pair OUT"=w7:T6)  [unwired: 8 in, 1 out]
  n2 = call "launch process event pair bag.vi"("launch items"=launch_items_list."pll engine", "bag action"=que_event_bag_action."check") -> ("even pair OUT"=w12:T6)  [unwired: 8 in, 1 out]
  n3 = Create User Event(user event datatype=w16) -> (user event=w15:refnum<user-event>)  [unwired: 1 in, 1 out]
  n4 = Unbundle By Name(w7) -> ("talkto event"=w6:refnum<user-event>)  [unwired: 1 out]
  n5 = Unbundle By Name(w12) -> ("talkto event"=w1:refnum<user-event>, "talkback event"=w14:refnum<user-event>)
  n6 = Create User Event(user event datatype=w20) -> (user event=w5:refnum<user-event>)  [unwired: 1 in, 1 out]
  n7 = Create User Event(user event datatype=w18) -> (user event=w13:refnum<user-event>)  [unwired: 1 in, 1 out]
  n8 = register-events(w5) -> (reference out=w23:refnum<event-registration>)  [unwired: 2 in, 1 out]
  n9 = register-events(w14, w15, w6) -> (reference out=w22:refnum<event-registration>)  [unwired: 2 in, 1 out]
  n10 = register-events(w13) -> (reference out=w17:refnum<event-registration>)  [unwired: 2 in, 1 out]
  n11 = control-ref of="Plot: complex plane"() -> (w21:refnum<vi>)
  n12 = call "freqgammabox.vi"("aggregator action"=agregator_--_action."init", "buffer size"=100) -> ("freq OUT (Hz)"=w2:dbl)  [unwired: 8 in, 1 out]
  n13 = while "communication Loop" {
    tunnel: w22 -> [w26]
    tunnel: w13 -> [w25]
    stop <- w24 stop-if-true
    n14 = event shown="[0] <talkback event>: User Event" {
      selector: w26 -> [_ _]
      dyn-events: _ -> [_ _]
      timeout: _ -> [_ _]
      tunnel: w25 -> [w27 w31]
      tunnel: [_ w32] -> w24
      event User Event {
        n15 = event-data() -> ("message"=w28:enum16{"new", "void"})  [unwired: 1 in]
        n16 = case shown="\"new\"" w28 {
          tunnel: w27 -> [_ w30]
          frame "void", Default {
          }
          frame "new" {
            n17 = Generate User Event(user event=w30, event data cluster="action: new" ("event data")) -> ()  [unwired: 2 in, 2 out]
          }
        }
      }
      event User Event {
        n18 = event-data() -> ("message"=w33:T11)  [unwired: 1 in]
        n19 = case shown="\"stop\", Default" w33 {
          tunnel: [_ TRUE] -> w32
          tunnel: w31 -> [_ w35]
          frame "stop", Default {
          }
          frame "exit" {
            w34 = "action: exit"  # action
            n20 = Generate User Event(user event=w35, event data cluster=w34) -> ()  [unwired: 2 in, 2 out]
          }
        }
      }
    }
  }
  n21 = while "interface Loop" {
    tunnel: w23 -> [w41]
    tunnel: w5 -> [w40]
    tunnel: w21 -> [w39]
    tunnel: w13 -> [w37]
    stop <- w38 stop-if-true
    n22 = event shown="[0] <interface>: User Event" {
      selector: w41 -> [_ _ _ _ _ _ _ _]
      dyn-events: _ -> [_ _ _ _ _ _ _ _]
      timeout: _ -> [_ _ _ _ _ _ _ _]
      tunnel: [_ "Toggle PLL :@" _ "Reset freq :r" "Reset lore :q" "reset from basic" "save lor for later" _] -> _
      tunnel: w40 -> [w44 w80 _ _ w116 _ _ w131]
      tunnel: w39 -> [w45 _ w86 _ _ _ _ w130]
      tunnel: [w43 _ _ _ _ _ _ _] -> w38
      tunnel: w37 -> [w42 _ _ w113 w118 _ _ w129]
      event User Event {
        n23 = event-data() -> ("interface"=w46:T10)  [unwired: 1 in]
        n24 = case shown="\"unpause pll\"" w46 {
          tunnel: w45 -> [_ _ _ _ _ _ w72 _]
          tunnel: w44 -> [_ _ _ _ _ w56 _ w74]
          tunnel: [_ _ _ _ TRUE _ _ _] -> w43
          tunnel: w42 -> [_ w47 w49 w52 _ _ _ _]
          frame "void", Default {
          }
          frame "pause pll" {
            w48 = "action: pause pll"  # action
            n25 = Generate User Event(user event=w47, event data cluster=w48) -> ()  [unwired: 2 in, 2 out]
          }
          frame "unpause pll" {
            w50 = "action: unpause pll"  # action
            n26 = Generate User Event(user event=w49, event data cluster=w50) -> ()  [unwired: 2 in, 2 out]
          }
          frame "start pll async" {
            n27 = Generate User Event(user event=w52, event data cluster="action: start pll async" ("event data")) -> ()  [unwired: 2 in, 2 out]
          }
          frame "exit" {
          }
          frame "toggle pll async" {
            n28 = local read "PLL is ON"() -> (w55:bool)
            n29 = case shown="False" w55 {
              tunnel: [pll_internal_user_event_action."unpause pll" ("event data") pll_internal_user_event_action."pause pll" ("event data")] -> w54
              frame False {
              }
              frame True {
              }
            }
            n30 = Generate User Event(user event=w56, event data cluster=w54) -> ()  [unwired: 2 in, 2 out]
          }
          frame "update cursors" {
            n31 = local read "lorentzian"() -> (w59:T2)
            n32 = Unbundle By Name(w59) -> ("4corners.z(inf)"=w67:cdb, "4corners.z(0)"=w60:cdb)
            n33 = Complex To Re/Im(x + iy=w67) -> (x=w69:dbl, y=w68:dbl)
            n34 = Complex To Re/Im(x + iy=w60) -> (x=w63:dbl, y=w62:dbl)
            n35 = call "replace cursor - plot ref - V2.vi"("Plot ref in"=w72, "new X"=w69, "new  Y"=w68, "cursor index"=2, "cursor action"=cursor_action."write", "Color Box"=u32 16746738) -> ()  [unwired: 10 in, 4 out]
            n36 = call "replace cursor - plot ref - V2.vi"("Plot ref in"=w72, "new X"=w63, "new  Y"=w62, "cursor index"=3, "cursor action"=cursor_action."write", "Color Box"=u32 10682154) -> ()  [unwired: 10 in, 4 out]
          }
          frame "toggle sweeper" {
            n37 = case shown="True" "PLL is ON" {
              tunnel: w74 -> [_ w76]
              frame False {
              }
              frame True {
                n38 = Generate User Event(user event=w76, event data cluster=pll_internal_user_event_action."pause pll" ("event data")) -> ()  [unwired: 2 in, 2 out]
              }
            }
            n39 = Generate User Event(user event=w74, event data cluster=pll_internal_user_event_action."start sweeper" ("event data")) -> ()  [unwired: 2 in, 2 out]
          }
        }
      }
      event "Toggle PLL :@": Value Change {
        w78 = pll_internal_user_event_action."toggle pll async"  # event data
        n40 = event-data() -> ()  [unwired: 1 in, 1 out]
        n41 = Generate User Event(user event=w80, event data cluster=w78) -> ()  [unwired: 2 in, 2 out]
      }
      event "Plot: complex plane": Cursor Move {
        n42 = event-data() -> ("CursIdx"=w85:i32)  [unwired: 1 in]
        n43 = local read "lorentzian"() -> (w84:T2)
        n44 = case shown="2" w85 {
          selector: w85 -> [_ w98 w108]
          tunnel: w86 -> [_ w92 w107]
          tunnel: w84 -> [w87 w88 w106]
          tunnel: [w87 w89 w103] -> w82
          frame 0, Default {
          }
          frame 2 {
            n45 = call "replace cursor - plot ref - V2.vi"("Plot ref in"=w92, "cursor index"=w98, "cursor action"=cursor_action."read") -> ("read X"=w100:dbl, "read Y"=w101:dbl)  [unwired: 13 in, 2 out]
            n46 = Re/Im To Complex(1:w101, 2:w100) -> (0:w99:cdb)
            n47 = Bundle By Name(cluster=w88, "bg (V)"=w99) -> (w97:T2)
            n48 = call "lorentzian transformations.vi"("4 corner circle transformation"=four-corner_circle_transformation."get4corners", "lorentzian in"=w97) -> ("lorentzian out"=w89:T2)  [unwired: 6 in, 3 out]
            n49 = Unbundle By Name(w89) -> ("4corners.z(0)"=w95:cdb)
            n50 = Complex To Re/Im(x + iy=w95) -> (x=w94:dbl, y=w93:dbl)
            n51 = call "replace cursor - plot ref - V2.vi"("Plot ref in"=w92, "new X"=w94, "new  Y"=w93, "cursor index"=3, "cursor action"=cursor_action."write") -> ()  [unwired: 11 in, 4 out]
          }
          frame 3 {
            n52 = call "replace cursor - plot ref - V2.vi"("Plot ref in"=w107, "cursor index"=w108, "cursor action"=cursor_action."read") -> ("read X"=w110:dbl, "read Y"=w111:dbl)  [unwired: 13 in, 2 out]
            n53 = Re/Im To Complex(1:w111, 2:w110) -> (0:w109:cdb)
            n54 = Bundle By Name(cluster=w106, "4corners.z(0)"=w109) -> (w105:T2)
            n55 = call "lorentzian transformations.vi"("4 corner circle transformation"=four-corner_circle_transformation."update lorentzian -- from z0", "lorentzian in"=w105) -> ("lorentzian out"=w103:T2)  [unwired: 6 in, 3 out]
          }
        }
        n56 = call "lorentzian transformations.vi"("4 corner circle transformation"=four-corner_circle_transformation."get4corners", "lorentzian in"=w82) -> ("lorentzian out"=w81:T2)  [unwired: 6 in, 3 out]
        n57 = local write "lorentzian"(w81) -> ()
      }
      event "Reset freq :r": Value Change {
        n58 = event-data() -> ()  [unwired: 1 in, 1 out]
        n59 = Generate User Event(user event=w113, event data cluster="action: accept frequency" ("event data")) -> ()  [unwired: 2 in, 2 out]
      }
      event "Reset lore :q": Value Change {
        n60 = event-data() -> ()  [unwired: 1 in, 1 out]
        n61 = Generate User Event(user event=w116, event data cluster=pll_internal_user_event_action."update cursors" ("event data")) -> ()  [unwired: 2 in, 2 out]
        n62 = Generate User Event(user event=w118, event data cluster="action: accept lorentzian" ("event data")) -> ()  [unwired: 2 in, 2 out]
      }
      event "reset from basic": Value Change {
        n63 = event-data() -> ()  [unwired: 1 in, 1 out]
        n64 = local read "lorentzian -- basic"() -> (w122:T2)
        n65 = call "lorentzian transformations.vi"("4 corner circle transformation"=four-corner_circle_transformation."get4corners", "lorentzian in"=w122) -> ("lorentzian out"=w121:T2)  [unwired: 6 in, 3 out]
        n66 = local write "lorentzian"(w121) -> ()
      }
      event "save lor for later": Value Change {
        n67 = event-data() -> ()  [unwired: 1 in, 1 out]
        n68 = local read "lorentzian"() -> (w126:T2)
        n69 = call "lorentzian transformations.vi"("4 corner circle transformation"=four-corner_circle_transformation."get4corners", "lorentzian in"=w126) -> ("lorentzian out"=w125:T2)  [unwired: 6 in, 3 out]
        n70 = local write "lorentzian -- basic"(w125) -> ()
      }
      event Key Down {
        n71 = event-data() -> ("Char"=w133:i16, "VKey"=w135:T14)  [unwired: 1 in]
        n72 = Build Array(w133) -> (w134:i16[])
        n73 = Byte Array To String(unsigned byte array=w134) -> (string=w132:string)
        n74 = case shown="\"ASCII\", Default" w135 {
          selector: w135 -> [_ _ _ _ w158]
          tunnel: w133 -> [_ _ _ _ _]
          tunnel: w132 -> [w139 _ _ _ _]
          tunnel: w131 -> [w138 _ _ _ _]
          tunnel: w130 -> [w137 _ _ _ w157]
          tunnel: w129 -> [w136 _ _ _ _]
          frame "ASCII", Default {
            n75 = case shown="\"q\"" w139 {
              selector: w139 -> [_ w141 _ _ _ _ _]
              tunnel: w138 -> [_ _ _ _ w151 w153 _]
              tunnel: w137 -> [_ w140 _ _ _ _ _]
              tunnel: w136 -> [_ _ w148 _ _ _ w155]
              frame "0", Default {
              }
              frame "<", ">", "?", "A", "z" {
                n76 = case shown="\"A\"" w141 {
                  tunnel: [cursor_action."zoom out 20%" ("cursor action") cursor_action."zoom in 20%" ("cursor action") cursor_action."smart zoom out&aspect" ("cursor action") cursor_action."smart zoom out" ("cursor action") cursor_action."zoom to aspect ratio 1" ("cursor action")] -> w142
                  frame ">" {
                  }
                  frame "<" {
                  }
                  frame "?" {
                  }
                  frame "A" {
                  }
                  frame "z", Default {
                  }
                }
                n77 = call "replace cursor - plot ref - V2.vi"("Plot ref in"=w140, "cursor action"=w142) -> ()  [unwired: 14 in, 4 out]
              }
              frame "r" {
                (unwired) pll_internal_user_event_action."accept frequency" ("event data")
                (unwired) "reset frequency" ("event data")
                n78 = Generate User Event(user event=w148, event data cluster="action: accept frequency" ("event data")) -> ()  [unwired: 2 in, 2 out]
              }
              frame "'", ";", "[", "]", "{", "}" {
              }
              frame "@" {
                (unwired) "toggle PLL" ("event data")
                n79 = Generate User Event(user event=w151, event data cluster=pll_internal_user_event_action."toggle pll async" ("event data")) -> ()  [unwired: 2 in, 2 out]
              }
              frame "#" {
                (unwired) "(sweeper) sweep!" ("event data")
                n80 = Generate User Event(user event=w153, event data cluster=pll_internal_user_event_action."toggle sweeper" ("event data")) -> ()  [unwired: 2 in, 2 out]
              }
              frame "q" {
                (unwired) pll_internal_user_event_action."accept lorentzian" ("event data")
                n81 = Generate User Event(user event=w155, event data cluster="action: accept lorentzian" ("event data")) -> ()  [unwired: 2 in, 2 out]
              }
            }
          }
          frame "Escape" {
          }
          frame "PageUp" {
          }
          frame "PageDown" {
          }
          frame "Up".."Right" {
            n82 = case shown="\"Down\"" w158 {
              tunnel: [cursor_action."move range right 20%" ("cursor action") cursor_action."move range left 20%" ("cursor action") cursor_action."move range up 20%" ("cursor action") cursor_action."move range down 20%" ("cursor action")] -> w156
              frame "Right", Default {
              }
              frame "Left" {
              }
              frame "Up" {
              }
              frame "Down" {
              }
            }
            n83 = call "replace cursor - plot ref - V2.vi"("Plot ref in"=w157, "cursor action"=w156) -> ()  [unwired: 14 in, 4 out]
          }
        }
      }
    }
  }
  n84 = while "action Loop" {
    tunnel: w17 -> [w167]
    tunnel: w13 -> [w165]
    tunnel: w5 -> [w164]
    tunnel: w1 -> [w163]
    stop <- w166 stop-if-true
    n85 = event shown="[0] <action>: User Event" {
      selector: w167 -> [_]
      dyn-events: _ -> [_]
      timeout: _ -> [_]
      tunnel: [w170] -> w166
      tunnel: w165 -> [_]
      tunnel: w164 -> [w169]
      tunnel: w163 -> [w168]
      event User Event {
        n86 = event-data() -> ("action"=w171:string)  [unwired: 1 in]
        n87 = case shown="\"action: accept frequency\"" w171 {
          tunnel: [_ _ _ _ _ _ TRUE] -> w170
          tunnel: w169 -> [_ _ _ _ _ _ w208]
          tunnel: w168 -> [_ w191 w198 w201 w203 w205 _]
          frame "action: new", Default {
            w181 = 0.0 ("new X")
            n88 = call "publish -- pll result.vi"("publisher action"=publisher_action."get") -> ("pll result OUT"=w188:T17)  [unwired: 10 in]
            n89 = Unbundle By Name(w188) -> ("freq (Hz)"=→"fast f (Hz)":dbl, "gamma (Hz)"=→"fast G (Hz)":dbl, "Voltage (V)"=w189:cdb, "running lorentzian out"=→"running lorentzian out":T2)
            "zi out (V)" <- w189
            n90 = Complex To Re/Im(x + iy=w189) -> (x=→"zi out Re (V)":dbl, y=→"zi out Im (V)":dbl)
            n91 = control-ref of="Plot: complex plane"() -> (w190:refnum<vi>)
            n92 = Complex To Re/Im(x + iy=w189) -> (x=w185:dbl, y=w184:dbl)
            n93 = call "replace cursor - plot ref - V2.vi"("Plot ref in"=w190, "new X"=w185, "new  Y"=w184, "cursor index"=0, "cursor action"=cursor_action."write", "Color Box"=u32 327424) -> ("Plot ref out"=w183:refnum<vi>)  [unwired: 10 in, 3 out]
            n94 = call "replace cursor - plot ref - V2.vi"("Plot ref in"=w183, "new X"=w181, "new  Y"=w181, "cursor index"=1, "cursor action"=cursor_action."write", "Color Box"=u32 5880319) -> ()  [unwired: 10 in, 4 out]
          }
          frame "action: accept lorentzian" {
            n95 = call "publish -- lorentzian.vi"("publisher action"=publisher_action."get") -> ("lorentzian OUT"=w195:T2)  [unwired: 10 in]
            n96 = call "lorentzian transformations.vi"("4 corner circle transformation"=four-corner_circle_transformation."get4corners", "lorentzian in"=w195) -> ("lorentzian out"=w196:T2)  [unwired: 6 in, 3 out]
            n97 = local write "lorentzian"(w196) -> ()
            n98 = Generate User Event(user event=w191, event data cluster=T16 {"message"=enum."update request"} ("event data")) -> ()  [unwired: 2 in, 2 out]
          }
          frame "action: pause pll" {
            n99 = local write "PLL is ON"(FALSE ("PLL ON")) -> ()
            n100 = Generate User Event(user event=w198, event data cluster=T16 {"message"=enum."pause"} ("event data")) -> ()  [unwired: 2 in, 2 out]
          }
          frame "action: unpause pll" {
            n101 = local write "PLL is ON"(TRUE ("PLL ON")) -> ()
            n102 = Generate User Event(user event=w201, event data cluster=T16 {"message"=enum."unpause"} ("event data")) -> ()  [unwired: 2 in, 2 out]
          }
          frame "action: start pll async" {
            n103 = Generate User Event(user event=w203, event data cluster=T16 {"message"=enum."start"} ("event data")) -> ()  [unwired: 2 in, 2 out]
          }
          frame "action: accept frequency" {
            n104 = Generate User Event(user event=w205, event data cluster=T16 {"message"=enum."reset"} ("event data")) -> ()  [unwired: 2 in, 2 out]
          }
          frame "action: exit" {
            n105 = Generate User Event(user event=w208, event data cluster=pll_internal_user_event_action."exit" ("event data")) -> ()  [unwired: 2 in, 2 out]
            n106 = local write "is publish loop stoped?"(TRUE ("Stoped?")) -> ()
            n107 = local write "PLL is ON"(FALSE ("PLL ON")) -> ()
          }
        }
      }
    }
  }
  n108 = while "publish Loop" {
    tunnel: w2 -> [_]
    stop <- w243 stop-if-true
    n109 = call "publish -- lorentzian.vi"("publisher action"=publisher_action."get") -> ("lorentzian OUT"=w212:T2)  [unwired: 10 in]
    "static lorentzian out" <- w212
    n110 = local read "average time (sec)"() -> (w228:dbl)
    n111 = local write "lorentzian"(w212) -> ()
    n112 = Multiply(x="publish dt (sec)", y=1000.0) -> (x*y=w241:dbl)
    n113 = Wait Until Next ms Multiple(millisecond multiple=w241) -> ()  [unwired: 1 out]
    n114 = Unbundle By Name(w212) -> ("f (Hz)"=w232:dbl, "G (Hz)"=w233:dbl)
    n115 = Divide(x=w228, y="publish dt (sec)") -> (x/y=w226:dbl)
    n116 = Round To Nearest(number=w226) -> (nearest integer value=w227:dbl)
    n117 = local read "fast G (Hz)"() -> (w218:dbl)
    n118 = local read "fast f (Hz)"() -> (w219:dbl)
    n119 = To Long Integer(number=w227) -> (32bit integer=w238:i32)
    n120 = case shown="True" TRUE {
      tunnel: [w249 w251] -> w234
      tunnel: [w248 w250] -> w235
      tunnel: w232 -> [w249 _]
      tunnel: w233 -> [w248 _]
      tunnel: w219 -> [_ w251]
      tunnel: w218 -> [_ w250]
      frame False {
      }
      frame True {
      }
    }
    n121 = local read "running lorentzian out"() -> (w214:T2)
    n122 = call "freqgammabox.vi"("aggregator action"=agregator_--_action."append", "buffer size"=w238, "Gamma (Hz)"=w235, "freq (Hz)"=w234) -> ("gamma OUT (Hz)"=w237:dbl, "freq OUT (Hz)"=w236:dbl)  [unwired: 6 in]
    n123 = call "freqgammabox.vi"("aggregator action"=agregator_--_action."interpolate", "buffer size"=w238, "Gamma (Hz)"=w237, "freq (Hz)"=w236) -> ("gamma OUT (Hz)"=w240:dbl, "freq OUT (Hz)"=w239:dbl)  [unwired: 6 in]
    "slow f (Hz)" <- w239
    "slow G (Hz)" <- w240
    n124 = Unbundle By Name(w212) -> ("4corners"=w213:T3)
    n125 = Unbundle By Name(w214) -> ("4corners"=w217:T3)
    n126 = call "draw complex lorentzian.vi"("4 corners"=w213) -> ("fancy circles"=w229:cluster{dbl[], dbl[]}[])  [unwired: 10 in]
    n127 = local read "zi out (V)"() -> (w220:cdb)
    n128 = Bundle By Name(cluster=T4 {"freq (Hz)"=0.0, "gamma (Hz)"=0.0, "Voltage (V)"=0.0+0.0i} ("publish message"), "freq (Hz)"=w239, "gamma (Hz)"=w240, "Voltage (V)"=w220) -> (w215:T4)
    "publish message" <- w215
    n129 = call "draw complex lorentzian.vi"("4 corners"=w217) -> ("fancy circles"=w230:cluster{dbl[], dbl[]}[])  [unwired: 10 in]
    n130 = Build Array (concatenate)(w229, w230) -> (→"Plot: complex plane":cluster{dbl[], dbl[]}[])
    n131 = Unbundle By Name(w215) -> ("freq (Hz)"=w246:dbl, "Voltage (V)"=w245:cdb, "gamma (Hz)"=w244:dbl)
    n132 = local read "is publish loop stoped?"() -> (w243:bool)
    n133 = call "publish -- get frequency and voltage.vi"("running lorentzian in"=w214, "publisher action"=publisher_action."set", "freq IN (Hz)"=w246, "static lorentzian IN"=w212, "Voltage IN (V)"=w245, "gamma IN (Hz)"=w244) -> ()  [unwired: 5 in, 5 out]
  }
  n134 = disable-structure shown="Disabled" {
    disable-tunnel: _ -> [w270 _]
    disable-tunnel: _ -> [w269 _]
    disable-tunnel: [w254 _] -> _
    disable-tunnel: _ -> [w252 _]
    frame Disabled {
      n135 = call "linear interp iiii- complex - z-omega.vi"("z"=w270, "omega"=w269) -> ("slope"=w268:cdb)  [unwired: 5 in, 8 out]
      n136 = Unbundle By Name(w252) -> ("4corners.z center"=w253, "A (VHz)"=w263, "G (Hz)"=w265)
      n137 = Complex To Polar(r * e^(i*theta)=w268) -> (r=w267:dbl)  [unwired: 1 out]
      n138 = Divide(x=w268, y=w267) -> (x/y=w266:cdb)
      n139 = Reciprocal(x=w265) -> (1/x=w264:dbl)
      n140 = Compound Arithmetic op=MULTIPLY(w266, w264, w263, 1.1 ("value")) -> (w256:cdb)
      n141 = Add(x=w253, y=w256) -> (x+y=w262:cdb)
      n142 = Subtract(x=w253, y=w256) -> (x-y=w261:cdb)
      n143 = Complex To Re/Im(x + iy=w262) -> (x=w260:dbl, y=w258:dbl)
      n144 = Complex To Re/Im(x + iy=w261) -> (x=w259:dbl, y=w257:dbl)
      n145 = call "draw a line.vi"("y1"=w257, "y0"=w258, "x1"=w259, "x0"=w260) -> ("output cluster"=w254:cluster{dbl[], dbl[]})  [unwired: 7 in]
    }
    frame Enabled {
    }
  }
  n146 = disable-structure shown="Disabled" {
    disable-tunnel: _ -> [w271 _]
    frame Disabled {
      n147 = call "lorentzian transformations.vi"("4 corner circle transformation"=four-corner_circle_transformation."get4corners", "lorentzian in"="lorentzian -- hist") -> ("4corners our"=w275:T3)  [unwired: 6 in, 3 out]
      n148 = Complex To Re/Im(x + iy=w271) -> (x=w278:dbl, y=w277:dbl)
      n149 = call "draw complex lorentzian.vi"("4 corners"=w275) -> ("fancy circles"=w273:cluster{dbl[], dbl[]}[])  [unwired: 10 in]
      n150 = Bundle(w278, w277) -> (w279:cluster{dbl, dbl})  [unwired: 1 in]
      n151 = Build Array (concatenate)(w279, w273) -> (→"Plot: complex- hist":cluster{dbl[], dbl[]}[])
    }
    frame Enabled {
    }
  }
  "is publish loop stoped?" <- FALSE ("Stoped?")
